vi "Configure Dialog.vi"(8 "error in (no error)":errorcluster, 11 "Abort Generation Msg in":refnum<class "Abort Generation Msg.lvclass">) -> (0 "error out":errorcluster, 2 "Ok?":bool, 3 "Abort Generation Msg out":refnum<class "Abort Generation Msg.lvclass">)   [LabVIEW 2014, in "CS++Fgen.lvlib" / "Abort Generation Msg.lvclass"]
uses:
  Abort Generation Msg.lvclass
  Abort Generation Msg.lvclass/Abort Generation Msg.ctl
panel:
  in  "Abort Button":bool
  in  "Cancel Button":bool
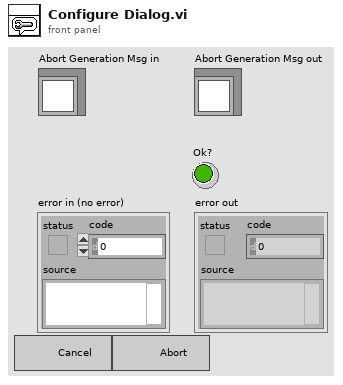
[diagram p1: front panel]
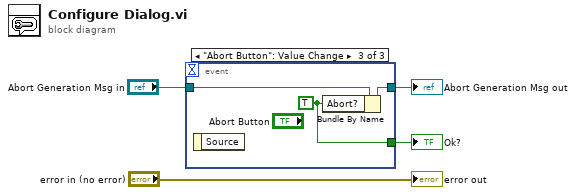
[diagram p0: block diagram]
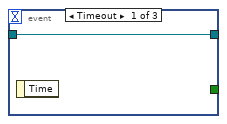
[diagram p2: hidden frame]
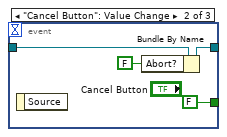
[diagram p3: hidden frame]
diagram:
  n1 = event shown="[2] \"Abort Button\": Value Change" {
    selector: _ -> [_ _ _]
    dyn-events: _ -> [_ _ _]
    timeout: _ -> [_ _ _]
    tunnel: [w5 w7 w11] -> w3
    tunnel: "Abort Generation Msg in" -> [w5 w9 w12]
    tunnel: [_ FALSE w10] -> w1
    event Timeout {
      n2 = event-data() -> ()  [unwired: 1 in, 1 out]
    }
    event "Cancel Button": Value Change {
      n3 = event-data() -> ()  [unwired: 1 in, 1 out]
      n4 = Bundle By Name(cluster=w9, "Abort?"=FALSE) -> (w7:refnum<class "Abort Generation Msg.lvclass">)
    }
    event "Abort Button": Value Change {
      w10 = TRUE ("Abort?")
      n5 = event-data() -> ()  [unwired: 1 in, 1 out]
      n6 = Bundle By Name(cluster=w12, "Abort?"=w10) -> (w11:refnum<class "Abort Generation Msg.lvclass">)
    }
  }
  "Abort Generation Msg out" <- w3
  "Ok?" <- w1
  "error out" <- "error in (no error)"
